vi "JSONConstants.vi"() -> ()   [LabVIEW 2017]
panel:
  out "IDName":string="ID"
  out "TypeName":string="Type"
  out "ComponentsName":string="Components"
  out "NIDocumentName":string="NIDocument"
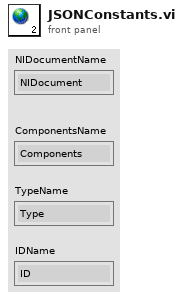
[diagram p1: front panel]
diagram:
